vi "MH_ClearHistMem.vi"(8 "error in (no error)":errorcluster, 11 "devidx":i32) -> (0 "error out":errorcluster, 3 "return type":i32)   [LabVIEW 2019]
uses:
  <userlib>/MultiHarp150/MH_DllPath_global.vi
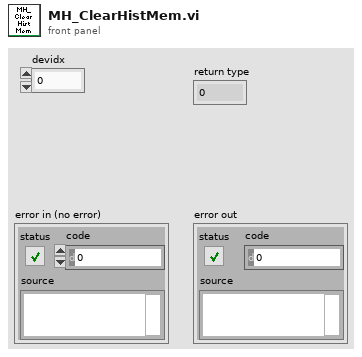
[diagram p1: front panel]
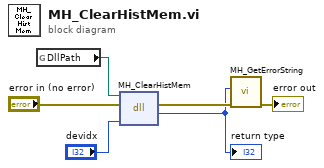
[diagram p0: block diagram]
diagram:
  n1 = global read "MH_DllPath_global.vi" "DllPath"() -> (w5:path)
  n2 = dll-call lib="MHLib64.dll" fn="MH_ClearHistMem"(path in=w5, error in="error in (no error)", "devidx"="devidx") -> (error out=w4:errorcluster, "return type"=w2:i32)  [unwired: 2 in, 1 out]
  "return type" <- w2
  n3 = call <userlib>:"MH_GetErrorString.vi"("error in (no error)"=w4, "code"=w2) -> ("error out"=→"error out":errorcluster)  [unwired: 7 in, 2 out]
